vi "Parse Multiline Basic String.vi"(8 "error in (no error)":errorcluster, 10 "start at":i32, 11 "TOML String":string) -> (0 "error out":errorcluster, 2 "offset past match":i32, 3 "String":string)   [LabVIEW 2017, in "TOML.lvlib"]
uses:
  TOML.lvlib
  <vilib>/Utility/error.llb/Error Cluster From Error Code.vi
  <vilib>/regexp/Match Regular Expression.xnode
  <vilib>/ErrorRing/Error Ring.xnode
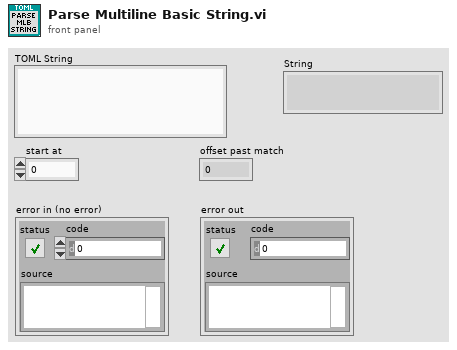
[diagram p1: front panel]
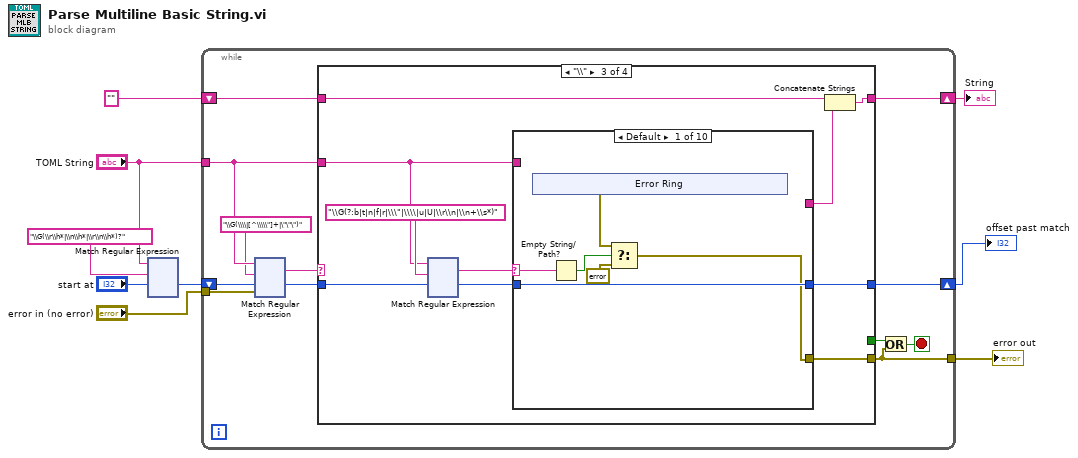
[diagram p0: block diagram]
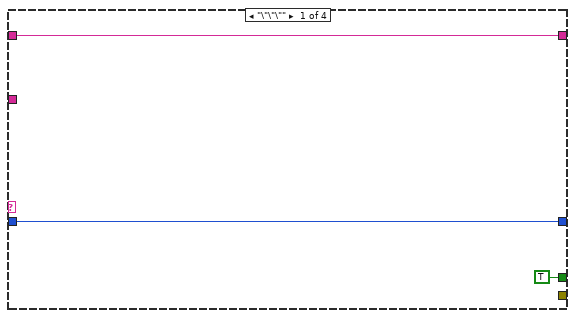
[diagram p2: hidden frame]
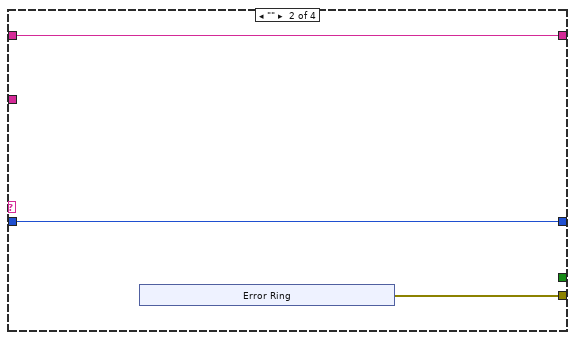
[diagram p3: hidden frame]
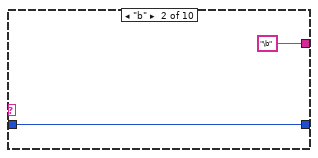
[diagram p4: hidden frame]
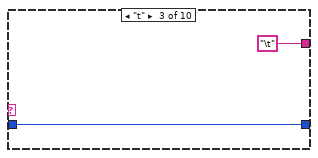
[diagram p5: hidden frame]
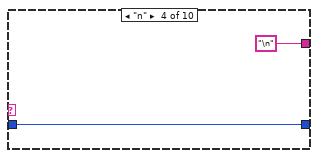
[diagram p6: hidden frame]
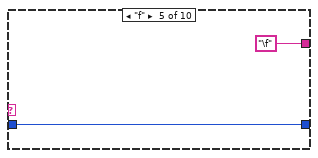
[diagram p7: hidden frame]
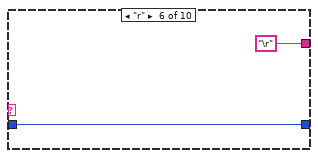
[diagram p8: hidden frame]
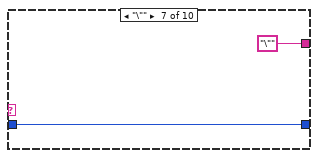
[diagram p9: hidden frame]
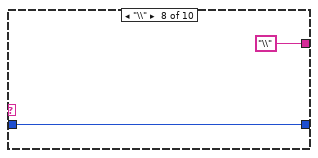
[diagram p10: hidden frame]
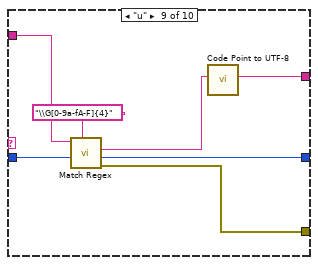
[diagram p11: hidden frame]
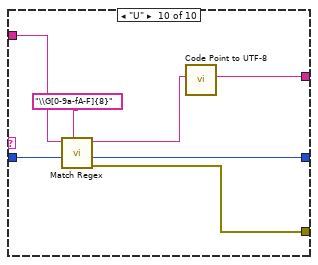
[diagram p12: hidden frame]
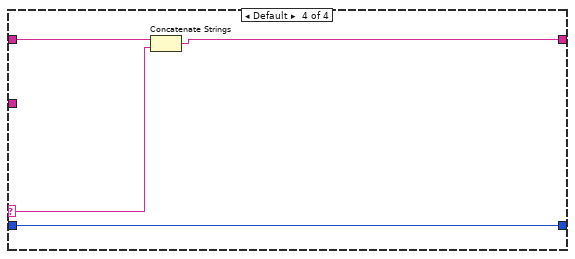
[diagram p13: hidden frame]
diagram:
  n1 = xnode "Match Regular Expression"("input string"="TOML String", "regular expression"="\\G(\\r\\h*|\\n\\h*|\\r\\n\\h*)?", "offset (0)"="start at") -> ("offset past match"=w3:i32)  [unwired: 3 in, 4 out]
  n2 = while {
    tunnel: "error in (no error)" -> [w21]
    tunnel: "TOML String" -> [w14]
    shift-right: [w19] -> w5
    shift-left: w3 -> [w20]
    shift-right: [w17] -> w6
    shift-left: "" -> [w16]
    tunnel: [w12] -> w7
    stop <- w13 stop-if-true
    n3 = xnode "Match Regular Expression"("input string"=w14, "regular expression"="\\G(\\\\|[^\\\\\"]+|\"\"\")", "offset (0)"=w20, "error in"=w21) -> ("whole match"=w11:string, "offset past match"=w18:i32)  [unwired: 2 in, 3 out]
    n4 = case shown="\"\\\\\"" w11 {
      selector: w11 -> [_ _ _ w196]
      tunnel: [w23 w26 w37 w197] -> w19
      tunnel: w18 -> [w23 w26 w40 w197]
      tunnel: [w24 w27 w35 w194] -> w17
      tunnel: w16 -> [w24 w27 w41 w195]
      tunnel: [TRUE _ _ _] -> w15
      tunnel: w14 -> [_ _ w33 _]
      tunnel: [_ w25 w38 _] -> w12
      frame "\"\"\"" {
      }
      frame "" {
        n5 = xnode "Error Ring"() -> ("error out"=w25:errorcluster)
      }
      frame "\\" {
        n6 = xnode "Match Regular Expression"("input string"=w33, "regular expression"="\\G(?:b|t|n|f|r|\\\"|\\\\|u|U|\\r\\n|\\n+\\s*)", "offset (0)"=w40) -> ("whole match"=w32:string, "offset past match"=w36:i32)  [unwired: 3 in, 3 out]
        n7 = case shown="Default" w32 {
          selector: w32 -> [w46 _ _ _ _ _ _ _ _ _]
          tunnel: [w43 _ _ _ _ _ _ _ w69 w75] -> w38
          tunnel: [w47 w52 w54 w56 w58 w60 w62 w64 w70 w76] -> w37
          tunnel: w36 -> [w47 w52 w54 w56 w58 w60 w62 w64 w71 w77]
          tunnel: [_ "\b" ("regular expression") "\t" ("regular expression") "\n" ("regular expression") "\f" ("regular expression") "\r" ("regular expression") "\"" ("regular expression") "\\" ("regular expression") w66 w73] -> w34
          tunnel: w33 -> [_ _ _ _ _ _ _ _ w72 w78]
          frame Default {
            n8 = xnode "Error Ring"() -> ("error out"=w42:errorcluster)
            n9 = Empty String/Path?(string/path=w46) -> (empty?=w45:bool)
            n10 = Select(t=w42, s=w45, f=errorcluster {"status"=FALSE, "code"=0, "source"=""}) -> (s? t:f=w43:errorcluster)
          }
          frame "b" {
          }
          frame "t" {
          }
          frame "n" {
          }
          frame "f" {
          }
          frame "r" {
          }
          frame "\"" {
          }
          frame "\\" {
          }
          frame "u" {
            n11 = call "Match Regex.vi"("regular expression"="\\G[0-9a-fA-F]{4}", "offset"=w71, "String"=w72) -> ("error out"=w69:errorcluster, "offset past match"=w70:i32, "submatch 1"=w67:string)  [unwired: 5 in, 1 out]
            n12 = call "Code Point to UTF-8.vi"("Code Point"=w67) -> ("UTF-8"=w66:string)  [unwired: 10 in]
          }
          frame "U" {
            n13 = call "Match Regex.vi"("regular expression"="\\G[0-9a-fA-F]{8}", "offset"=w77, "String"=w78) -> ("error out"=w75:errorcluster, "offset past match"=w76:i32, "whole match"=w74:string)  [unwired: 5 in, 1 out]
            n14 = call "Code Point to UTF-8.vi"("Code Point"=w74) -> ("UTF-8"=w73:string)  [unwired: 10 in]
          }
        }
        n15 = Concatenate Strings(w41, w34) -> (w35:string)
      }
      frame Default {
        n16 = Concatenate Strings(w195, w196) -> (w194:string)
      }
    }
    n17 = Or(x=w15, y=w12) -> (x .or. y?=w13:bool)
  }
  "error out" <- w7
  "offset past match" <- w5
  "String" <- w6
